vi "Calculate-POI x-axis value.vi"(5 "Total number of points in indexed ROI over the full experiment time":i32, 9 "Header Data":T1={"Number of POI"=0, "Number of Miniscans"=0, "Number of Trials"=0, "Number of Cycles "=0, "# Averaged Frames"=0, "Laser power (%)"=0, "Pockels"=0.0, "Acquisition Length (sec)"=0.0, "Fill time (us)"=0.0, "DwellTime (us)"=0.0, "Miniscan Dwell time per pixel (us)"=0.0, "PMT 1"=0.0, "PMT 2"=0.0, "Back Apperture"=0.0, "Zoom"=0.0, "Number of Pixels in Miniscan"=0, "Frame Size"=200, "Field of View"=0.0, "X centre"=0.0, "Y centre"=0.0, "AOL Z"=0.0} {"Frame Size" items=["100X100"=100, "128X128"=128, "200X200"=200, "256X256"=256, "512X512"=512, "1024x1024"=1024, "2048x2048"=2048]; "Back Apperture" format="%#.6g"; "Pockels" format="%#.6g"; "PMT 2" format="%#.6g"; "PMT 1" format="%#.6g"; "Miniscan Dwell time per pixel (us)" format="%#.6g"; "Zoom" format="%#.6g"; "DwellTime (us)" format="%#.6g"; "Acquisition Length (sec)" format="%#.6g"; "Fill time (us)" format="%#.6g"}, 10 "[ROI Time(us)]":dbl[](array[numeric]), 11 "ROI number":i32=1) -> (1 "POI X-axis values array (sec)":sgl[](array[numeric]) format="%#.9f")   [LabVIEW 2020]
uses:
  Experiment header interface/Typedefs/Header parameters cluster-Zstack.ctl
  Typedefs/Frame Size.ctl
panel:
  # "Zstack header parameters"
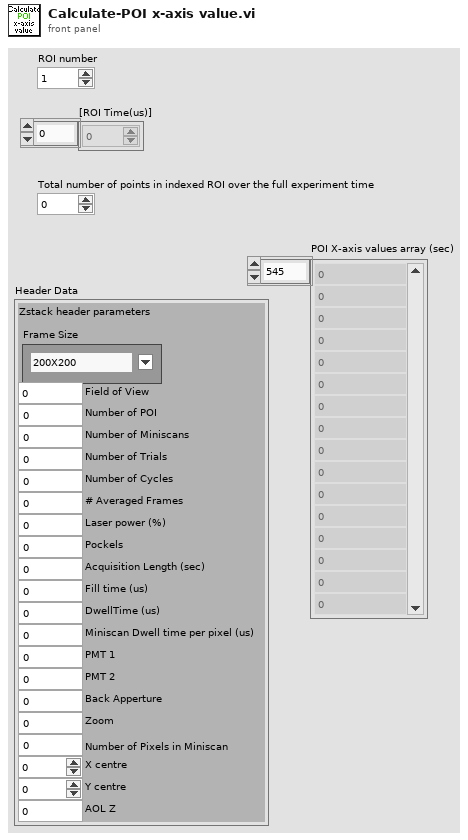
[diagram p1: front panel]
types:
  T1 = typedef "Header parameters cluster-Zstack.ctl" = cluster{"Number of POI":u16, "Number of Miniscans":u16, "Number of Trials":u16, "Number of Cycles ":u16, "# Averaged Frames":u16, "Laser power (%)":u8, "Pockels":dbl, "Acquisition Length (sec)":dbl, "Fill time (us)":dbl, "DwellTime (us)":dbl, "Miniscan Dwell time per pixel (us)":dbl, "PMT 1":dbl, "PMT 2":dbl, "Back Apperture":dbl, "Zoom":dbl, "Number of Pixels in Miniscan":u16, "Frame Size":T2, "Field of View":dbl, "X centre":dbl, "Y centre":dbl, "AOL Z":dbl}
  T2 = typedef "Frame Size.ctl" = u16
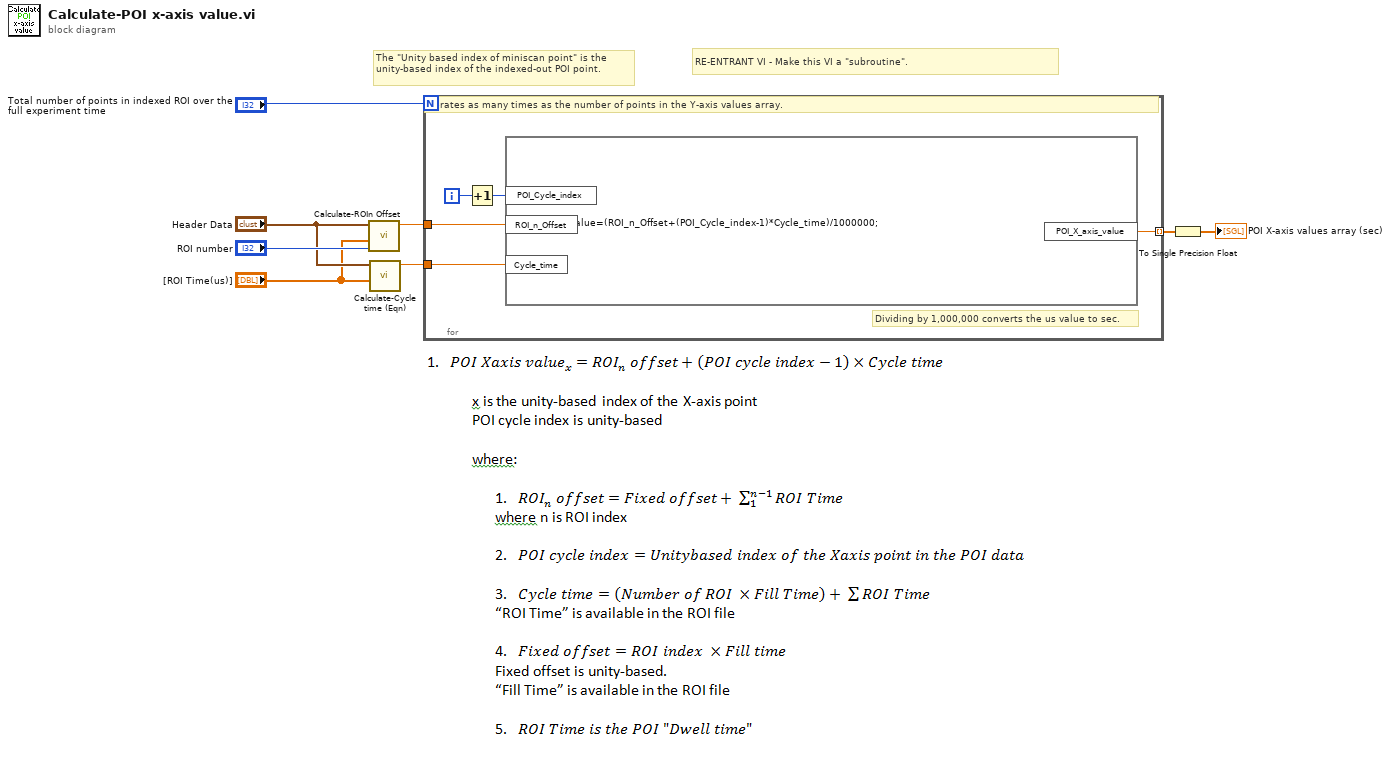
[diagram p0: block diagram]
diagram:
  # "RE-ENTRANT VI - Make this VI a \"subroutine\"."
  # "The \"Unity based index of miniscan point\" is the unity-based index of the indexed-out POI point."
  n1 = call "Calculate-ROIn Offset.vi"("ROI number"="ROI number", "[ROI Time(us)]"="[ROI Time(us)]", "Header data"="Header Data") -> ("ROI n Offset (us)"=w4:dbl)  [unwired: 8 in]
  n2 = call "Calculate-Cycle time (Eqn).vi"("[ROI Time (us)]"="[ROI Time(us)]", "Header data"="Header Data") -> ("Cycle Time (us)"=w5:dbl)  [unwired: 9 in]
  n3 = for {
    N: "Total number of points in indexed ROI over the full experiment time" -> [_]
    tunnel: [w13] -> w2 mode=indexing
    tunnel: w5 -> [w12]
    tunnel: w4 -> [w11]
    i -> [w10]
    # "Dividing by 1,000,000 converts the us value to sec."
    # "Iterates as many times as the number of points in the Y-axis values array."
    n4 = Increment(x=w10) -> (x+1=w9:i32)
    n5 = formula code="POI_X_axis_value=(ROI_n_Offset+(POI_Cycle_index-1)*Cycle_time)/1000000;"("POI_Cycle_index"=w9, "ROI_n_Offset"=w11, "Cycle_time"=w12) -> ("POI_X_axis_value"=w13:dbl)
  }
  n6 = To Single Precision Float(number=w2) -> (single precision float=→"POI X-axis values array (sec)":sgl[])
